vi "Publisher.vi"() -> ()   [LabVIEW 2022 SP3]
uses:
  <vilib>/LabVIEW Open Source Project/MQTT Client/Client class/Client.lvclass/Client.ctl
  <vilib>/LabVIEW Open Source Project/MQTT Connection/MQTT_Base/Base Class/MQTT_Base.lvclass/MQTT_Base.ctl
  <vilib>/LabVIEW Open Source Project/MQTT Websockets Connection/MQTT_Websockets/Connection/WebsocketsConnection.lvclass
  C:/Program Files/National Instruments/LabVIEW 2022/vi.lib/LabVIEW Open Source Project/Connection/Connection/Connection.lvclass
  <vilib>/LabVIEW Open Source Project/MQTT Client/Client class/Client.lvclass
  C:/Program Files/National Instruments/LabVIEW 2022/vi.lib/LabVIEW Open Source Project/MQTT Connection/MQTT_Base/Base Class/MQTT_Base.lvclass
  <vilib>/LabVIEW Open Source Project/MQTT Control Packets/Control Packets/PUBLISH/PUBLISH.lvclass
  <vilib>/LabVIEW Open Source Project/MQTT Connection/MQTT_Base/Base Class/MQTT_Base.lvclass
panel:
  in  "Period (ms)":i32
  in  "Connection":bool
  in  "Stop Client":bool
  out "Published":bool
  out "Waveform Chart":dbl(graph)
  out "last error":errorcluster
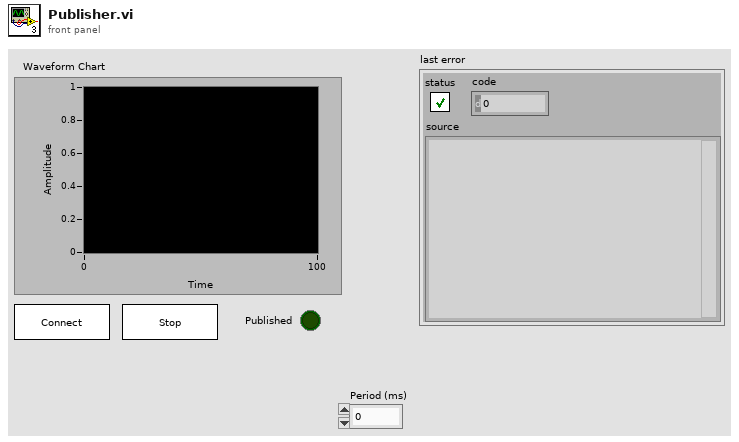
[diagram p1: front panel]
types:
  T1 = typedef "MQTT Client.lvlib/Client.lvclass/Public Events -- cluster.ctl" = cluster{"Connection Status":refnum<user-event>, "Connected":refnum<user-event>, "Application Message":refnum<user-event>}
  T2 = typedef "MQTT Base.lvlib/MQTT_Base.lvclass/Public Events -- cluster.ctl" = cluster{"Stop Event":refnum<user-event>, "Error Event":refnum<user-event>, "Inbound Message":refnum<user-event>}
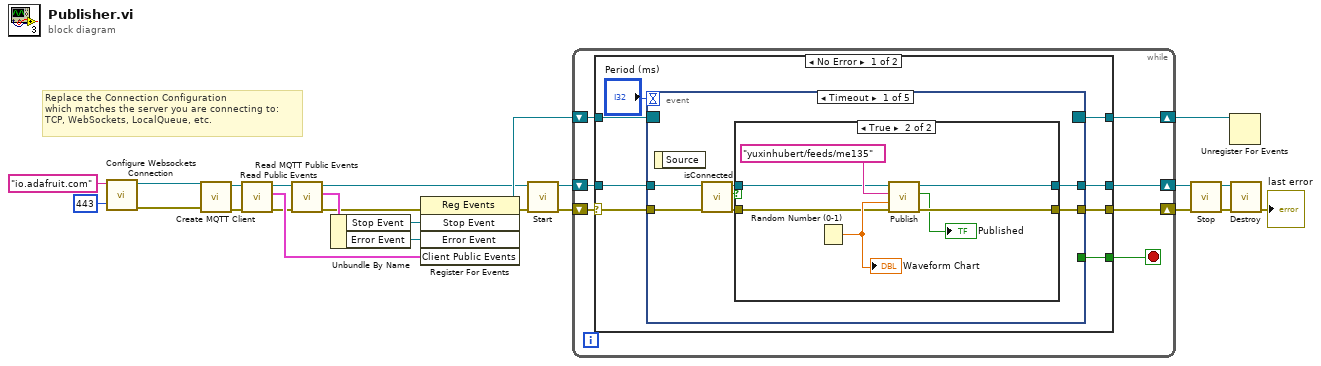
[diagram p0: block diagram]
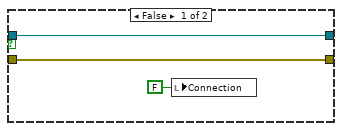
[diagram p2: hidden frame]
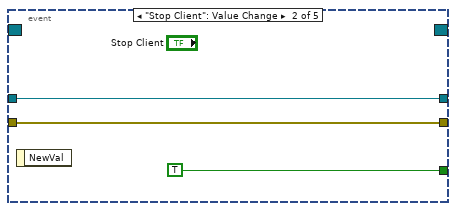
[diagram p3: hidden frame]
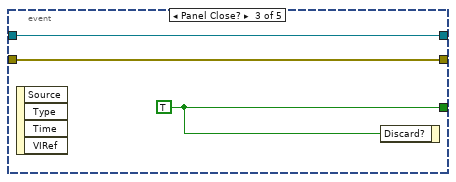
[diagram p4: hidden frame]
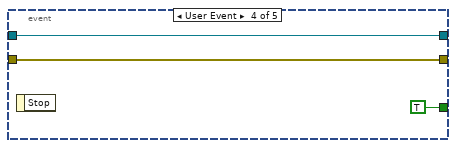
[diagram p5: hidden frame]
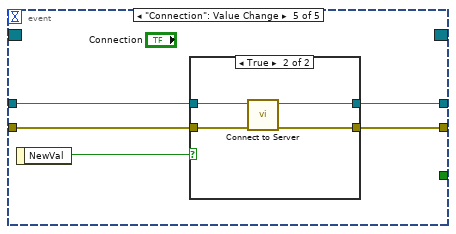
[diagram p6: hidden frame]
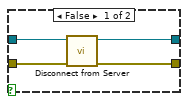
[diagram p7: hidden frame]
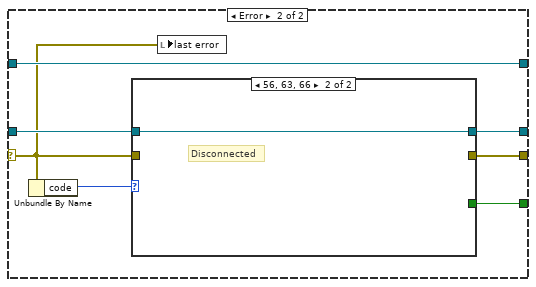
[diagram p8: hidden frame]
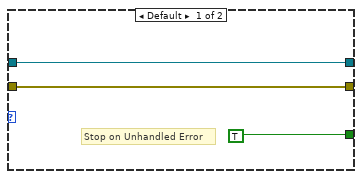
[diagram p9: hidden frame]
diagram:
  # "Replace the Connection Configuration\nwhich matches the server you are connecting to:\nTCP, WebSockets, LocalQueue, etc."
  n1 = call <vilib>:"Configure Websockets Connection.vi"("remote port (80)"=u16 443, "address (localhost)"="io.adafruit.com") -> ("error out"=w1:errorcluster, "WSConnection"=w2:refnum<class "WebsocketsConnection.lvclass">)  [unwired: 8 in]
  n2 = call <vilib>:"Create MQTT Client.vi"("error in (no error)"=w1, "Connection Configuration"=w2) -> ("error out"=w7:errorcluster, "Client out"=w5:refnum<class "Client.lvclass">)  [unwired: 8 in]
  n3 = call <vilib>:"Read Public Events.vi"("error in (no error)"=w7, "Client in"=w5) -> ("error out"=w8:errorcluster, "Client Public Events"=w10:T1, "Client out"=w6:refnum<class "Client.lvclass">)  [unwired: 7 in]
  n4 = call <vilib>:"Read MQTT Public Events.vi"("error in (no error)"=w8, "MQTT_Base in"=w6) -> ("error out"=w9:errorcluster, "MQTT Public Events"=w17:T2, "MQTT_Base out"=w12:refnum<class "Client.lvclass">)  [unwired: 7 in]
  n5 = Unbundle By Name(w17) -> ("Stop Event"=w15:refnum<user-event>, "Error Event"=w16:refnum<user-event>)
  n6 = register-events(error in=w9, w15, w16, w10) -> (reference out=w13:refnum<event-registration>, error out=w11:errorcluster)  [unwired: 1 in]
  n7 = call <vilib>:"Start.vi"("error in (no error)"=w11, "MQTT_Base in"=w12) -> ("error out"=w23:errorcluster, "MQTT_Base out"=w22:refnum<class "Client.lvclass">)  [unwired: 7 in, 1 out]
  n8 = while {
    shift-right: [w30] -> w14
    shift-left: w13 -> [w31]
    shift-right: [w27] -> w19
    shift-left: w22 -> [w28]
    shift-right: [w29] -> w21
    shift-left: w23 -> [w25]
    stop <- w26 stop-if-true
    n9 = case shown="No Error" w25 {
      selector: w25 -> [w33 w79]
      tunnel: w31 -> [w39 w85]
      tunnel: [w38 w85] -> w30
      tunnel: [w37 w81] -> w29
      tunnel: w28 -> [w36 w83]
      tunnel: [w35 w82] -> w27
      tunnel: [w34 w80] -> w26
      frame No Error {
        n10 = event shown="[0] Timeout" {
          selector: w39 -> [_ _ _ _ _]
          dyn-events: [_ _ _ _ _] -> w38
          timeout: "Period (ms)" -> [_ _ _ _ _]
          tunnel: w33 -> [w42 w58 w60 w65 w66]
          tunnel: [w45 w58 w60 w65 w67] -> w37
          tunnel: [_ TRUE w62 TRUE _] -> w34
          tunnel: w36 -> [w44 w59 w61 w63 w70]
          tunnel: [w46 w59 w61 w63 w68] -> w35
          event Timeout {
            n11 = event-data() -> ()  [unwired: 1 in, 1 out]
            n12 = call <vilib>:"isConnected.vi"("error in (no error)"=w42, "Client in"=w44) -> ("error out"=w41:errorcluster, "connected"=w40:bool, "Client out"=w43:refnum<class "Client.lvclass">)  [unwired: 7 in]
            n13 = case shown="True" w40 {
              tunnel: [w49 w55] -> w46
              tunnel: [w48 w54] -> w45
              tunnel: w43 -> [w49 w51]
              tunnel: w41 -> [w48 w50]
              frame False {
                n14 = local write "Connection"(FALSE ("Connection")) -> ()
              }
              frame True {
                n15 = Random Number (0-1)() -> (number: 0 to 1=w52:dbl)
                "Waveform Chart" <- w52
                n16 = call <vilib>:"Publish.vi"("error in (no error)"=w50, "Payload"=w52, "Topic Name (empty: Payload name)"="yuxinhubert/feeds/me135", "Client in"=w51) -> ("error out"=w54:errorcluster, "Published"=→"Published":bool, "Client out"=w55:refnum<class "Client.lvclass">)  [unwired: 5 in]
              }
            }
          }
          event "Stop Client": Value Change {
            n17 = event-data() -> ()  [unwired: 1 in, 1 out]
          }
          event Panel Close? {
            w62 = TRUE
            n18 = event-data() -> ()  [unwired: 1 in, 4 out]
            n19 = event-data("Discard?"=w62) -> ()  [unwired: 1 in, 1 out]
          }
          event User Event {
            n20 = event-data() -> ()  [unwired: 1 in, 1 out]
          }
          event "Connection": Value Change {
            n21 = event-data() -> ("NewVal"=w69:bool)  [unwired: 1 in]
            n22 = case shown="True" w69 {
              tunnel: w70 -> [w74 w78]
              tunnel: [w73 w75] -> w68
              tunnel: [w72 w76] -> w67
              tunnel: w66 -> [w71 w77]
              frame False {
                n23 = call <vilib>:"Disconnect from Server.vi"("error in (no error)"=w71, "Client in"=w74) -> ("error out"=w72:errorcluster, "Client out"=w73:refnum<class "Client.lvclass">)  [unwired: 7 in, 1 out]
              }
              frame True {
                n24 = call <vilib>:"Connect to Server.vi"("error in (no error)"=w77, "Client in"=w78) -> ("error out"=w76:errorcluster, "Client out"=w75:refnum<class "Client.lvclass">)  [unwired: 6 in, 2 out]
              }
            }
          }
        }
      }
      frame Error {
        n25 = Unbundle By Name(w79) -> ("code"=w84:i32)
        n26 = case shown="56, 63, 66" w84 {
          tunnel: w83 -> [w88 w89]
          tunnel: [w88 w89] -> w82
          tunnel: w79 -> [w87 _]
          tunnel: [w87 _] -> w81
          tunnel: [TRUE _] -> w80
          frame Default {
            # "Stop on Unhandled Error"
          }
          frame 56, 63, 66 {
            # "Disconnected"
          }
        }
        n27 = local write "last error"(w79) -> ()
      }
    }
  }
  n28 = call <vilib>:"Stop.vi"("error in (no error)"=w21, "MQTT_Base in"=w19) -> ("error out"=w20:errorcluster, "MQTT_Base out"=w18:refnum<class "Client.lvclass">)  [unwired: 7 in, 1 out]
  n29 = Unregister For Events(event registration refnum=w14) -> ()  [unwired: 1 in, 1 out]
  n30 = call <vilib>:"Destroy.vi"("error in (no error)"=w20, "MQTT_Base in"=w18) -> ("error out"=→"last error":errorcluster)  [unwired: 8 in, 1 out]
